vi "stop.vi"(8 "error in (no error)":errorcluster, 11 "DAQmx_pulse_out in":refnum<class "DAQmx_pulse_out.lvclass">) -> (0 "error out":errorcluster, 3 "DAQmx_pulse_out out":refnum<class "DAQmx_pulse_out.lvclass">)   [LabVIEW 2013, in "DAQmx_pulse_out.lvclass"]
uses:
  DAQmx_pulse_out.lvclass
  DAQmx_pulse_out.lvclass/DAQmx_pulse_out.ctl
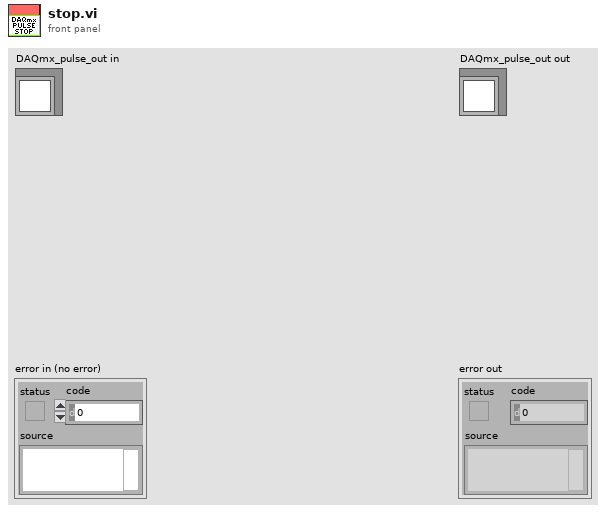
[diagram p1: front panel]
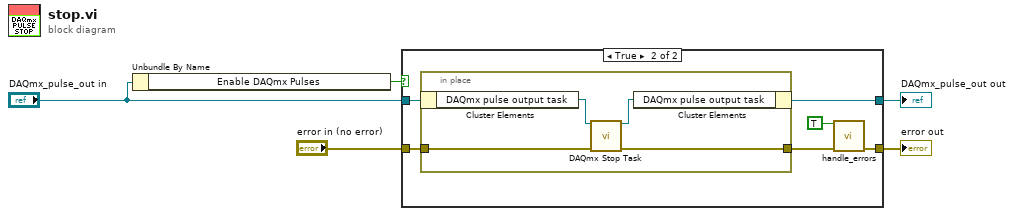
[diagram p0: block diagram]
diagram:
  n1 = Unbundle By Name("DAQmx_pulse_out in") -> ("Enable DAQmx Pulses"=w3:bool)
  n2 = case shown="True" w3 {
    tunnel: "error in (no error)" -> [w7 w13]
    tunnel: [w7 w11] -> w4
    tunnel: "DAQmx_pulse_out in" -> [w6 w9]
    tunnel: [w6 w8] -> w1
    frame False {
    }
    frame True {
      n3 = in-place {
        in-place-border: w13 -> [w17]
        in-place-border: [w16] -> w12
        n4 = in-place-cluster #1(w9) -> ("DAQmx pulse output task"=w15:refnum<k21>)
        n5 = call <vilib>:"DAQmx Stop Task.vi"("task/channels in"=w15, "error in"=w17) -> ("task out"=w14:refnum<k21>, "error out"=w16:errorcluster)  [unwired: 12 in]
        n6 = in-place-cluster #1("DAQmx pulse output task"=w14) -> (w8:refnum<class "DAQmx_pulse_out.lvclass">)
      }
      n7 = call "handle_errors.vi"("Exit Measurement"=TRUE, "error in (no error)"=w12) -> ("error out"=w11:errorcluster)  [unwired: 13 in]
    }
  }
  "error out" <- w4
  "DAQmx_pulse_out out" <- w1
